vi "oax_Generate Phase Modulated Signal.vi"(6 "init phase":dbl, 7 "fs":dbl, 8 "phase":dbl, 9 "order":dbl, 10 "time period":dbl[](array[numeric]), 11 "speed":dbl[](array[numeric])) -> (3 "y":dbl[](array[numeric]), 4 "final phase":dbl)   [LabVIEW 2017]
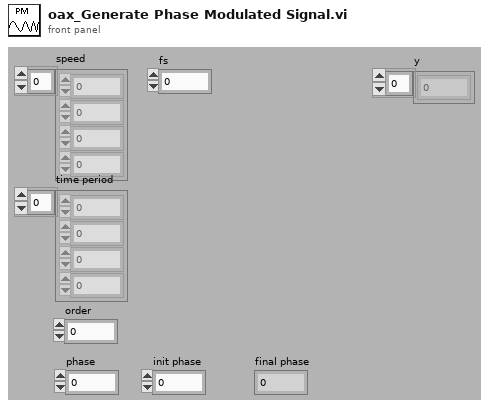
[diagram p1: front panel]
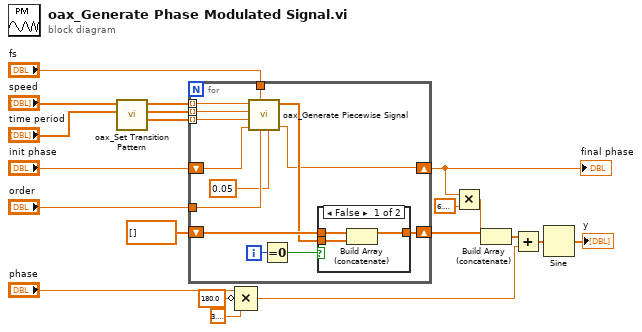
[diagram p0: block diagram]
diagram:
  n1 = call <vilib>:"oax_Set Transition Pattern.vi"("time period"="time period", "speed"="speed") -> ("time period"=w10:dbl[], "end speed"=w11:dbl[], "start speed/constant speed"=w12:dbl[])  [unwired: 7 in]
  n2 = for {
    tunnel: "order" -> [w33]
    tunnel: "fs" -> [w32]
    shift-right: [w28] -> w4
    shift-left: dbl[] [] ("speed 2") -> [w31]
    tunnel: w10 -> [w27] mode=indexing
    shift-right: [w24] -> w2
    shift-left: "init phase" -> [w23]
    tunnel: w12 -> [w22] mode=indexing
    tunnel: w11 -> [w21] mode=indexing
    i -> [w30]
    n3 = call <vilib>:"oax_Generate Piecewise Signal.vi"("acc transition ratio"=0.05, "order"=w33, "fs"=w32, "init phase"=w23, "time period"=w27, "end speed"=w21, "start speed/constant speed"=w22) -> ("final phase"=w24:dbl, "phase out"=w25:dbl[])  [unwired: 3 in]
    n4 = Equal To 0?(x=w30) -> (x = 0?=w29:bool)
    n5 = case shown="False" w29 {
      tunnel: w25 -> [w35 w37]
      tunnel: w31 -> [w36 _]
      tunnel: [w34 w37] -> w28
      frame False {
        n6 = Build Array (concatenate)(w36, w35) -> (w34:dbl[])
      }
      frame True {
      }
    }
  }
  "final phase" <- w2
  n7 = Compound Arithmetic op=MULTIPLY("phase", invert 180.0 ("value"), 3.141592653589793) -> (w7:dbl)
  n8 = Multiply(x=w2, y=6.283185307179586) -> (x*y=w1:dbl)
  n9 = Build Array (concatenate)(w4, w1) -> (w3:dbl[])
  n10 = Add(x=w3, y=w7) -> (x+y=w19:dbl[])
  n11 = Sine(x=w19) -> (sin(x)=→"y":dbl[])
